vi "Inline Replace.vi"(7 "Prevent Overwrite? (F)":bool, 8 "error in (no error)":errorcluster, 9 "renamed keys":string[](array[string]), 10 "keys":string[](array[string]), 11 "uData in":refnum<class "uData.lvclass">) -> (0 "error out":errorcluster, 1 "replaced?":bool[](array[boolean]), 2 "Found?":bool[](array[boolean]), 3 "uData out":refnum<class "uData.lvclass">)   [LabVIEW 2023, in "uLib.lvlib" / "uData.lvclass"]
doc: "Dynamic dispatch method to perform an inline replace operation.\n\n<B>THE \"INLINE\" DYNAMIC DISPATCH METHOD GROUP ARE THE ONLY METHODS THAT ARE ALLOWED TO ACCESS THE OBJECT PRIVATE DATA.</B>\n\nCONVERTED TO INLINE STATIC DISPATCH TO MITIGATE THE PERFORMANCE OVERHEAT HIT REALIZED IN INTIAL TESTING."
uses:
  uData.lvclass
  uData.lvclass/uData.ctl
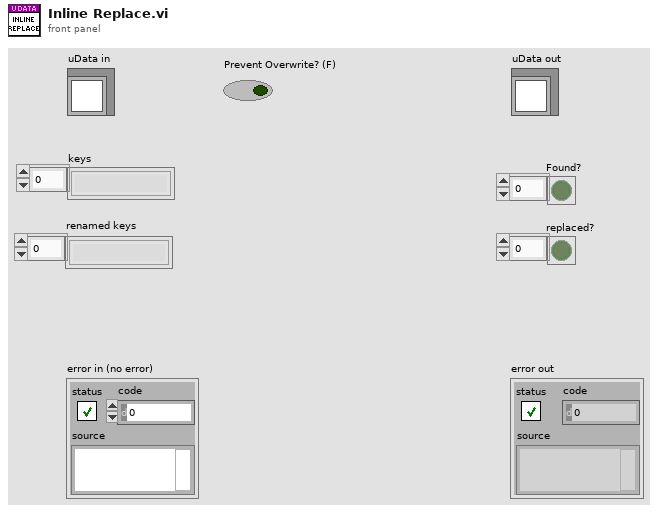
[diagram p1: front panel]
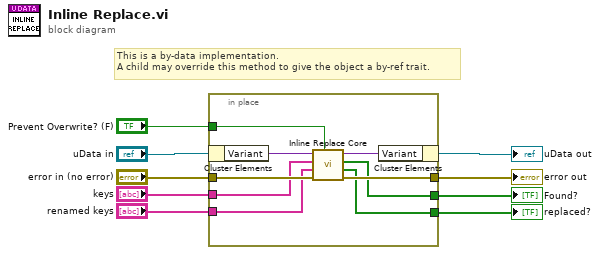
[diagram p0: block diagram]
diagram:
  # "This is a by-data implementation.\nA child may override this method to give the object a by-ref trait."
  n1 = in-place {
    in-place-border: [w15] -> w5
    in-place-border: "error in (no error)" -> [w16]
    in-place-border: [w12] -> w9
    in-place-border: "keys" -> [w13]
    in-place-border: "renamed keys" -> [w14]
    in-place-border: [w11] -> w2
    in-place-border: "Prevent Overwrite? (F)" -> [w10]
    n2 = in-place-cluster #1("uData in") -> ("Variant"=w18:variant)
    n3 = call "Inline Replace Core.vi"("Prevent Overwrite? (F)"=w10, "error in (no error)"=w16, "renamed keys"=w14, "keys"=w13, "Variant in"=w18) -> ("error out"=w15:errorcluster, "replaced?"=w12:bool[], "Found?"=w11:bool[], "Variant out"=w17:variant)  [unwired: 3 in]
    n4 = in-place-cluster #1("Variant"=w17) -> (→"uData out":refnum<class "uData.lvclass">)
  }
  "error out" <- w5
  "replaced?" <- w9
  "Found?" <- w2
